vi "Stop Timing Module.vi"(8 "error in (no error)":errorcluster, 10 "Structure Names":string, 11 "command":T1) -> (0 "error out":errorcluster)   [LabVIEW 2019]
uses:
  Stop Timing Module commands.vi
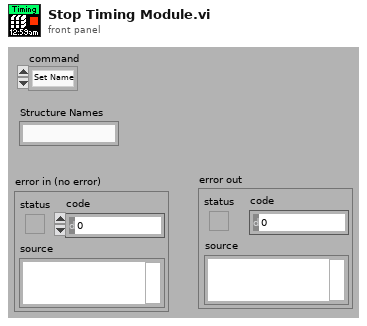
[diagram p1: front panel]
types:
  T1 = typedef "Stop Timing Module commands.vi" = enum16{"Set Name", "Stop loops"}
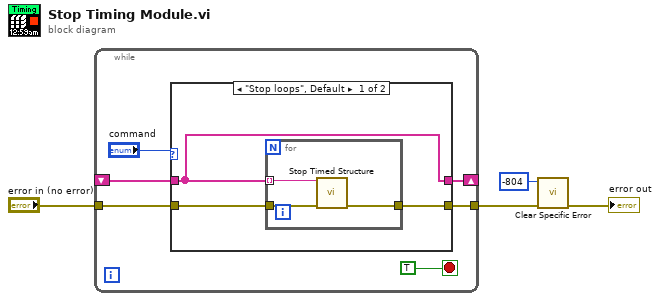
[diagram p0: block diagram]
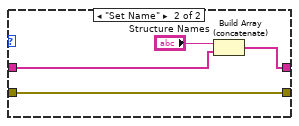
[diagram p2: hidden frame]
diagram:
  n1 = while {
    shift-right: [w8] -> _
    shift-left: _ -> [w7]
    tunnel: [w6] -> w2
    tunnel: "error in (no error)" -> [w5]
    stop <- TRUE stop-if-true
    n2 = case shown="\"Stop loops\", Default" "command" {
      tunnel: [w13 w18] -> w8
      tunnel: w7 -> [w13 w17]
      tunnel: [w12 w20] -> w6
      tunnel: w5 -> [w11 w20]
      frame "Stop loops", Default {
        n3 = for {
          tunnel: w13 -> [w16] mode=indexing
          tunnel: [w15] -> w12
          tunnel: w11 -> [w14]
          n4 = call <vilib>:"Stop Timed Structure.vi"("error in (no error)"=w14, "name"=w16) -> ("error out"=w15:errorcluster)  [unwired: 9 in]
        }
      }
      frame "Set Name" {
        n5 = Build Array (concatenate)("Structure Names", w17) -> (w18:string[])
      }
    }
  }
  n6 = call "Clear Specific Error.vi"("error in (no error)"=w2, "Code"=-804) -> ("error out"=→"error out":errorcluster)  [unwired: 5 in]
